vi "DisplayPanel.vi"() -> ()   [LabVIEW 2013]
uses:
  MvLVLib/MvCameraControl.lvlib
  <vilib>/picture/picture.llb/imagedata.ctl
panel:
  out "GenTLDevInfoArray":T1(array[cluster])
  out "GenTLIfInfoArray":T2(array[cluster])
  in  "Refresh Interaces":bool
  in  "Interface List":u16(ring) items=["[GenTL] GEVMV-GE1004-K88888888-100"]
  in  "pConvertInfo In":T3
  out "PixelFormat":u32
  out "handle out":u64
  in  "handle":u64
  in  "Rectangle":T4
  in  "image data":T5 caption="图像数据"
  out "Picture":picture
  out "PayloadSize":u32
  out "pFrameInfoEx out":T6
  out "nHeight":u32
  out "nWidth":u32
  out "Acquisision Flag":bool
  in  "Trigger Mode":bool
  in  "Continuous":bool
  out "打开标志":bool
  in  "stop":bool
  in  "Trigger Once":bool
  in  "Stop":bool
  in  "Start":bool
  in  "Open Device":bool
  in  "Close Device":bool
  in  "error in (no error) 2":errorcluster caption="错误输入（无错误）"
  in  "Refresh Devices":bool
  in  "Device List":u16(ring) items=["[GenTL]  MV-CA050-20GM(00598551000)"]
  # "Initialize"
  # "Acquisition"
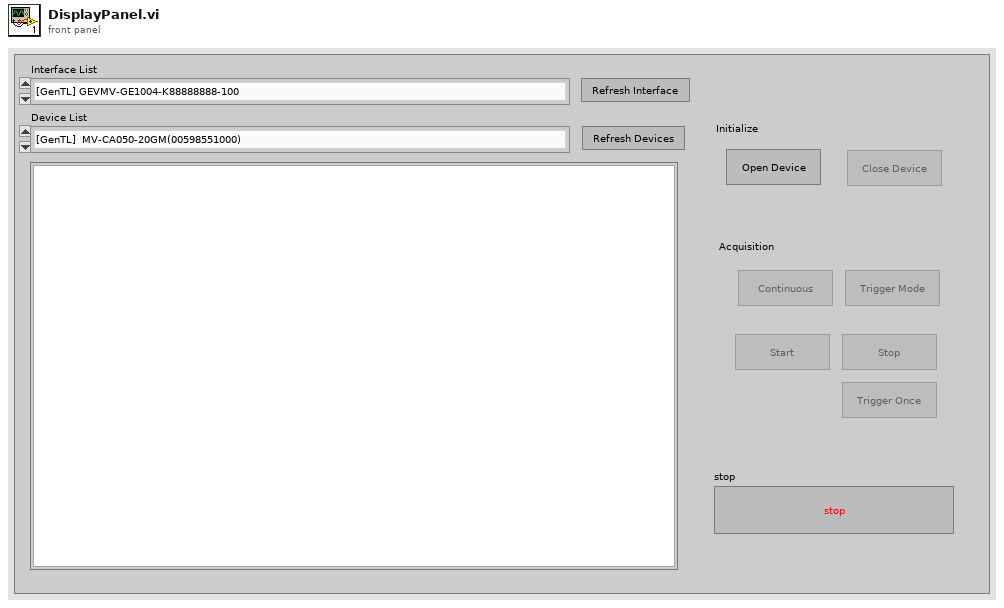
[diagram p1: front panel]
types:
  T1 = cluster{"chInterfaceID":string, "chDeviceID":string, "chVendorName":string, "chModelName":string, "chTLType":string, "chDisplayName":string, "chUserDefinedName":string, "chSerialNumber":string, "chDeviceVersion":string, "nCtiIndex":u32, "nReserved[0]":u32, "nReserved[1]":u32, "nReserved[2]":u32, "nReserved[3]":u32, "nReserved[4]":u32, "nReserved[5]":u32, "nReserved[6]":u32, "nReserved[7]":u32}[]
  T2 = cluster{"chInterfaceID":string, "chTLType":string, "chDisplayName":string, "nCtiIndex":u32, "nReserved[0]":u32, "nReserved[1]":u32, "nReserved[2]":u32, "nReserved[3]":u32, "nReserved[4]":u32, "nReserved[5]":u32, "nReserved[6]":u32, "nReserved[7]":u32}[]
  T3 = cluster{"nWidth":u16, "nHeight":u16, "enSrcPixelType":u32, "nSrcDataLen":u32, "enDstPixelType":u32, "nDstLen":u32, "nDstBufferSize":u32, "nRes0":u32, "nRes1":u32, "nRes2":u32, "nRes3":u32}
  T4 = cluster{"left":i16, "top":i16, "right":i16, "bottom":i16}
  T5 = typedef "imagedata.ctl" = cluster{"image type":i32, "image depth":i32, "image":u8[], "mask":u8[], "colors":u32[], "Rectangle":cluster{"left":i16, "top":i16, "right":i16, "bottom":i16}}
  T6 = cluster{"nWidth":u16, "nHeight":u16, "enPixelType":i32, "nFrameNum":u32, "nDevTimeStampHigh":u32, "nDevTimeStampLow":u32, "nReserved0":u32, "nHostTimeStamp":i64, "nFrameLen":u32, "nSecondCount]":u32, "nCycleCount":u32, "nCycleOffset":u32, "fGain":u32, "fExposureTime":u32, "nAverageBrightness":u32, "nRed":u32, "nGreen":u32, "nBlue":u32, "nFrameCounter":u32, "nTriggerIndex":u32, "nInput":u32, "nOutput":u32, "nOffsetX":u32, "nOffsetY":u32, "nReserved[0]":u32, "nReserved[1]":u32, "nReserved[2]":u32, "nReserved[3]":u32, "nReserved[4]":u32, "nReserved[5]":u32, "nReserved[6]":u32, "nReserved[7]":u32, "nReserved[8]":u32, "nReserved[9]":u32, "nReserved[10]":u32, "nReserved[11]":u32, "nReserved[12]":u32, "nReserved[13]":u32, "nReserved[14] 10":u32, "nReserved[15] 11":u32, "nReserved[16] 12":u32, "nReserved[17] 13":u32, "nReserved[18] 14":u32, "nReserved[19] 15":u32, "nReserved[20] 16":u32, "nReserved[21] 17":u32, "nReserved[22] 18":u32, "nReserved[23] 19":u32, "nReserved[24] 20":u32, "nReserved[25] 21":u32, "nReserved[26] 22":u32, "nReserved[27] 23":u32, "nReserved[28] 24":u32, "nReserved[29] 25":u32, "nReserved[30] 26":u32, "nReserved[31] 27":u32, "nReserved[32] 28":u32, "nReserved[33] 29":u32, "nReserved[34] 30":u32, "nReserved[35] 31":u32, "nReserved[36] 32":u32, "nReserved[37] 33":u32, "nReserved[38] 34":u32, "nReserved[39] 35":u32, "nReserved[40] 36":u32}
  T7 = enum8{"Enabled", "Disabled", "Disabled and Grayed Out"}
  T8 = cluster{"chInterfaceID":string, "chTLType":string, "chDisplayName":string, "nCtiIndex":u32, "nReserved[0]":u32, "nReserved[1]":u32, "nReserved[2]":u32, "nReserved[3]":u32, "nReserved[4]":u32, "nReserved[5]":u32, "nReserved[6]":u32, "nReserved[7]":u32}
  T9 = cluster{"chInterfaceID":string, "chDeviceID":string, "chVendorName":string, "chModelName":string, "chTLType":string, "chDisplayName":string, "chUserDefinedName":string, "chSerialNumber":string, "chDeviceVersion":string, "nCtiIndex":u32, "nReserved[0]":u32, "nReserved[1]":u32, "nReserved[2]":u32, "nReserved[3]":u32, "nReserved[4]":u32, "nReserved[5]":u32, "nReserved[6]":u32, "nReserved[7]":u32}
  T10 = cluster{"nCurValue":u32, "nMax":u32, "nMin":u32, "nInc":u32, "nReserved[0]":u32, "nReserved[1]":u32, "nReserved[2]":u32, "nReserved[3]":u32}
  T11 = cluster{"nCurValue":u32, "nSupportedNum":u32, "nSupportValue":u32[], "nReserved[0]":u32, "nReserved[1]":u32, "nReserved[2]":u32, "nReserved[3]":u32}
  T12 = cluster{"nWidth":u32, "nHeight":u32, "enSrcPixelType":u32, "nSrcDataLen":u32, "enDstPixelType":u32, "nDstLen":u32, "nDstBufferSize":u32, "nRes0":u32, "nRes1":u32, "nRes2":u32, "nRes3":u32}
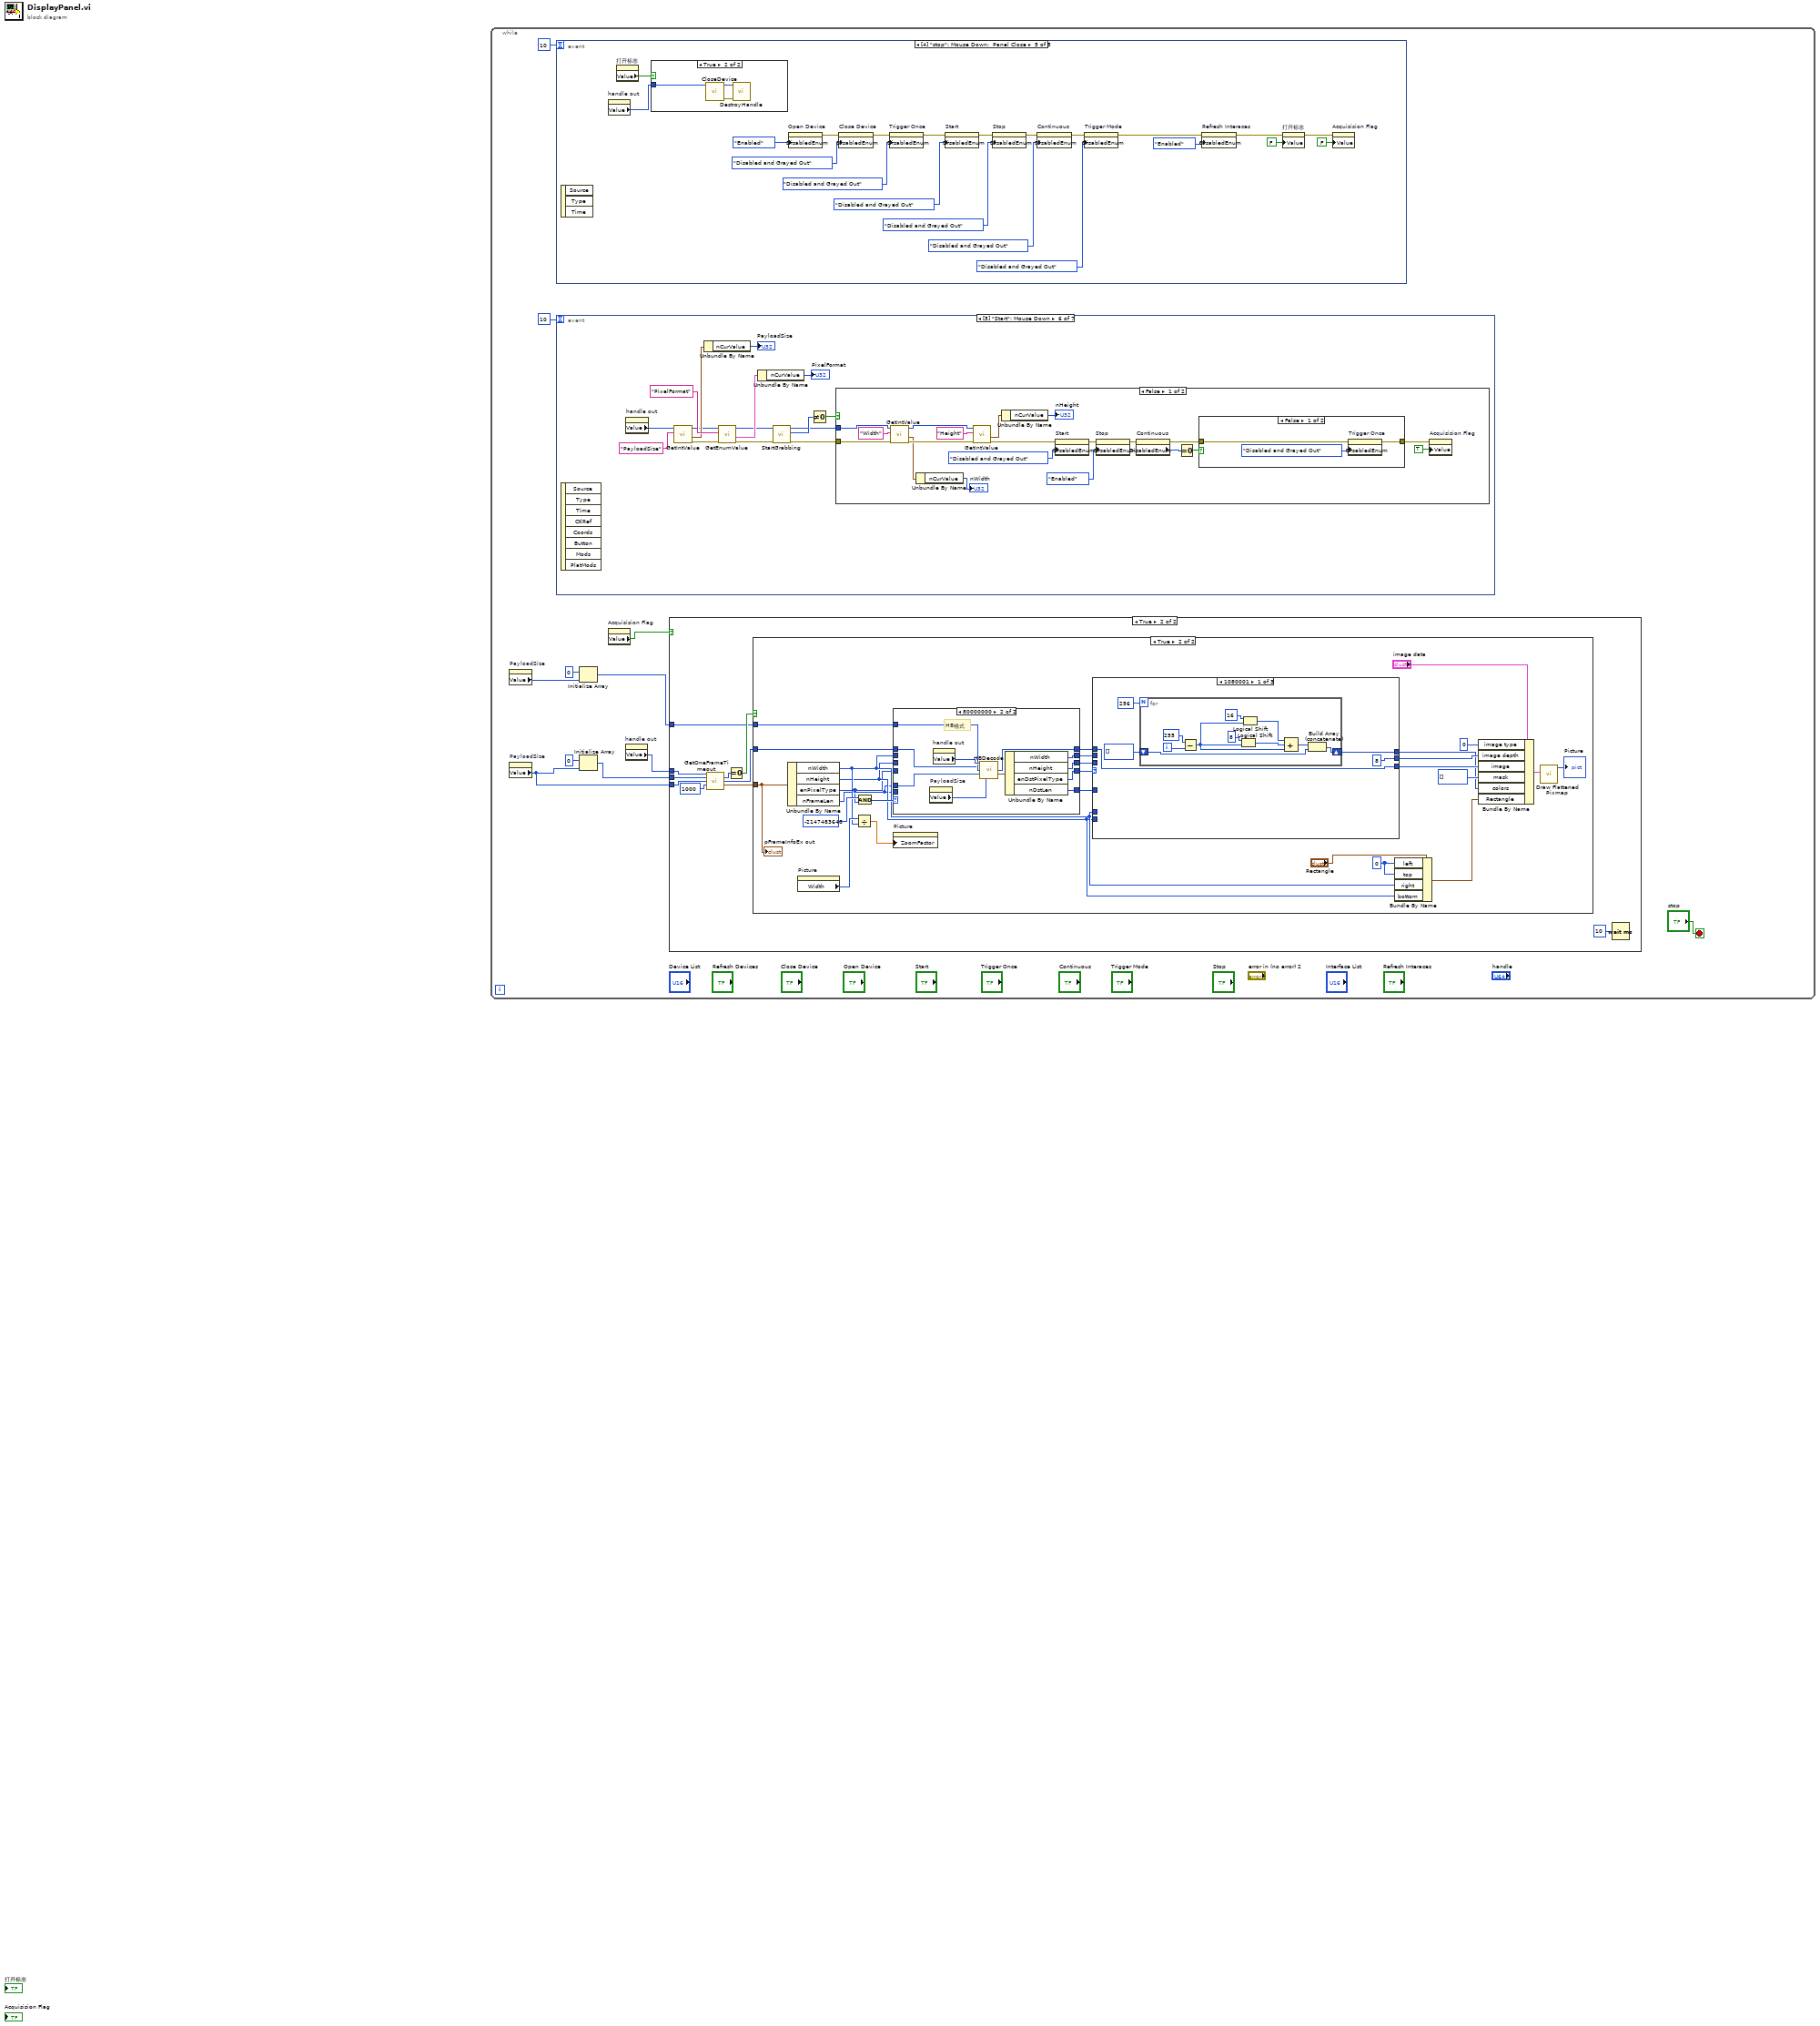
[diagram p0: block diagram]
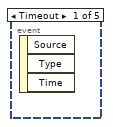
[diagram p2: hidden frame]
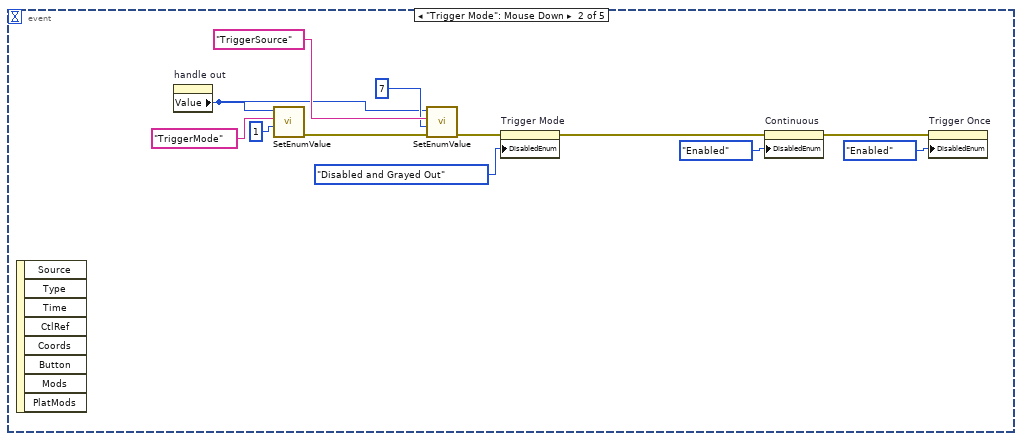
[diagram p3: hidden frame]
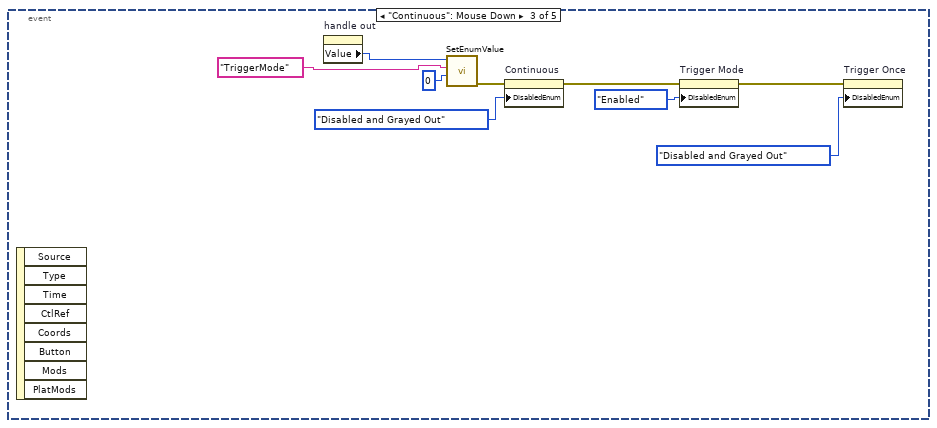
[diagram p4: hidden frame]
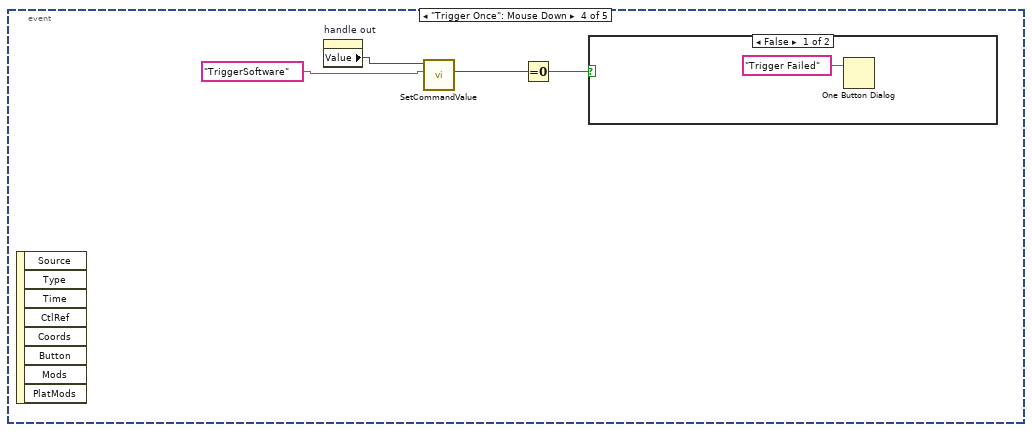
[diagram p5: hidden frame]
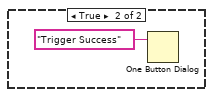
[diagram p6: hidden frame]
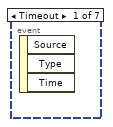
[diagram p8: hidden frame]
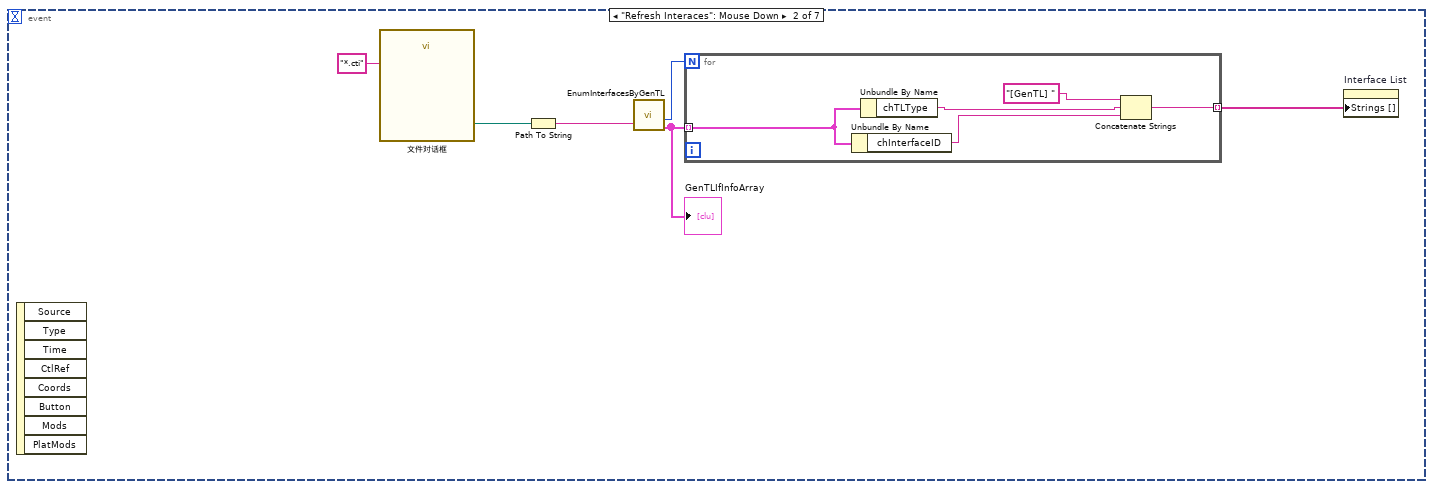
[diagram p9: hidden frame]
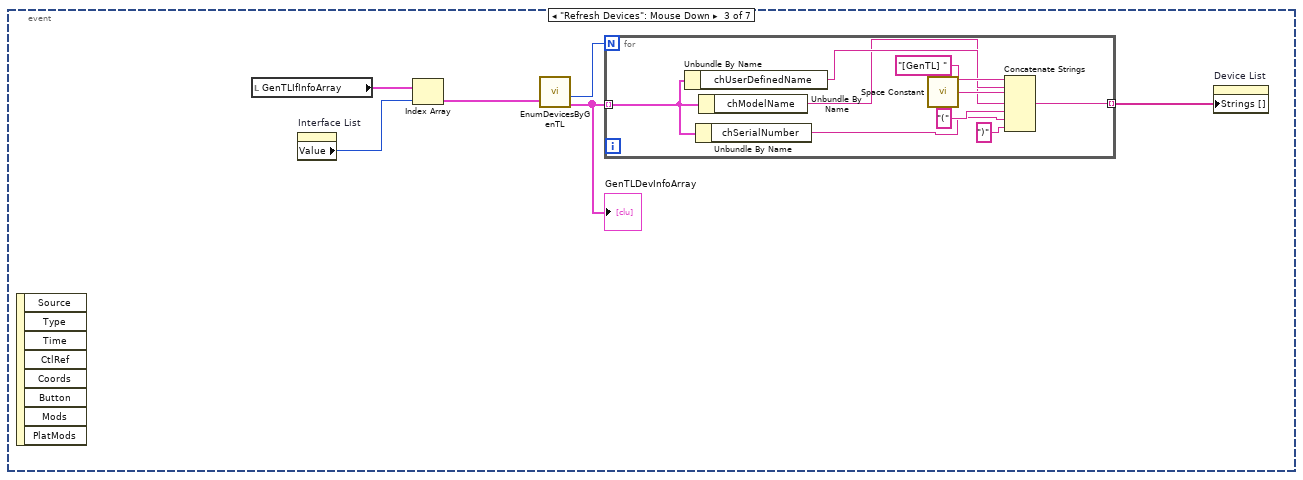
[diagram p10: hidden frame]
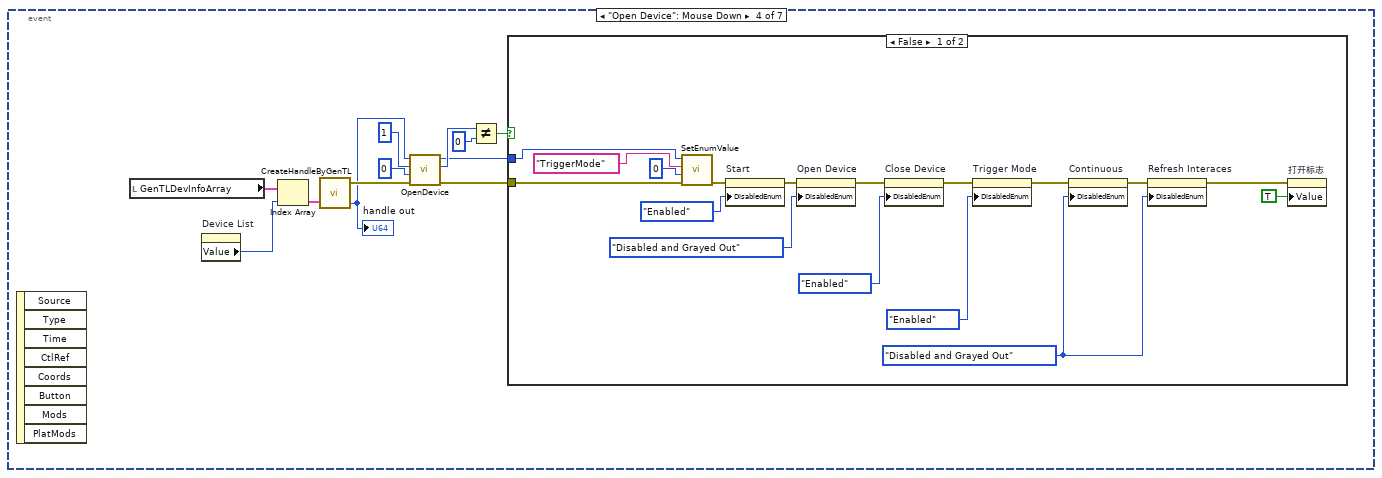
[diagram p11: hidden frame]
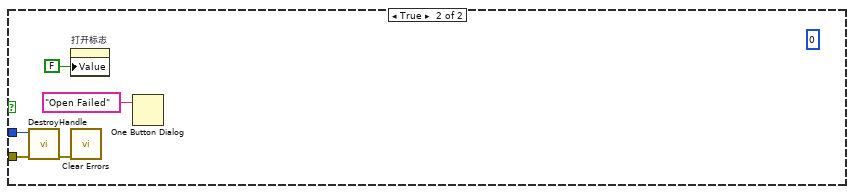
[diagram p12: hidden frame]
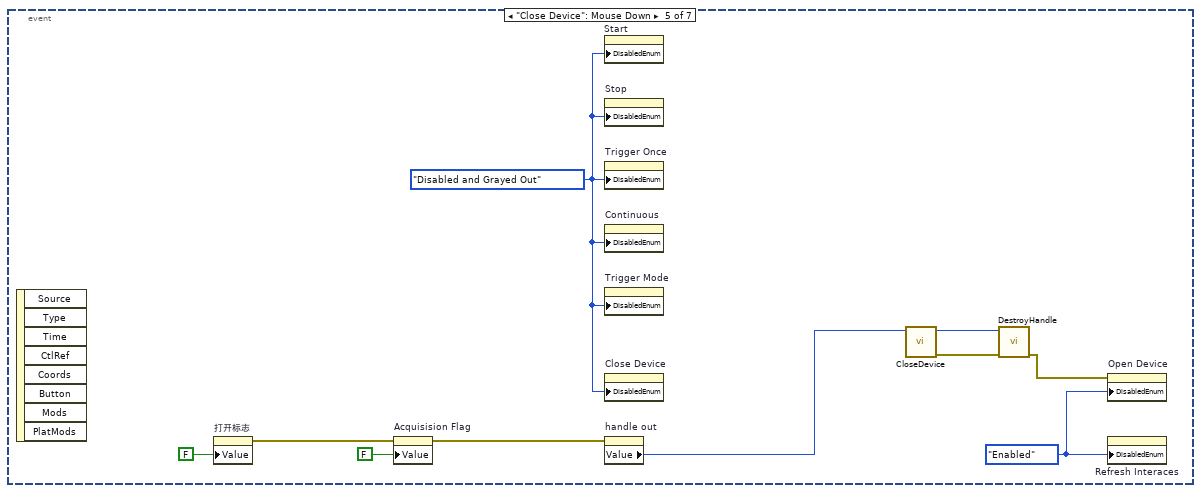
[diagram p13: hidden frame]
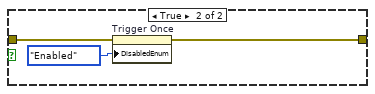
[diagram p14: hidden frame]
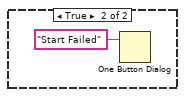
[diagram p15: hidden frame]
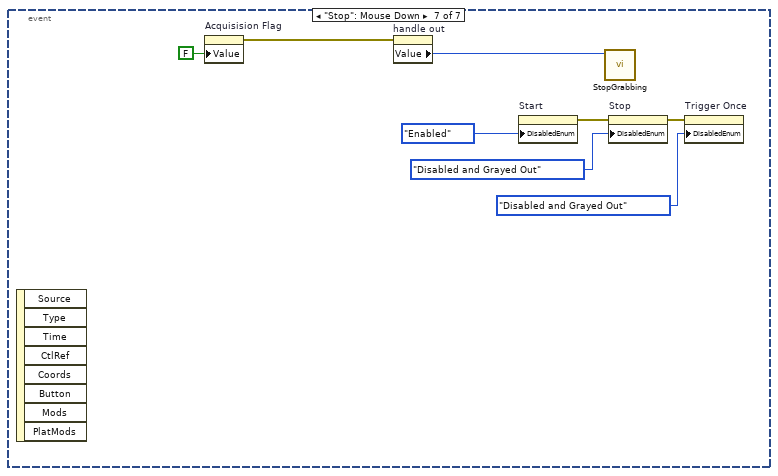
[diagram p16: hidden frame]
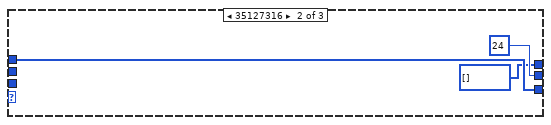
[diagram p20: hidden frame]
diagram:
  n1 = while {
    stop <- "stop" stop-if-true
    n2 = property on="PayloadSize" class="DigNum (strict)"() -> ("Value"=w5:u32)  [unwired: 2 in, 2 out]
    n3 = property on="PayloadSize" class="DigNum (strict)"() -> ("Value"=w6:u32)  [unwired: 2 in, 2 out]
    n4 = event shown="[4] \"stop\": Mouse Down;  Panel Close" {
      selector: _ -> [_ _ _ _ _]
      dyn-events: _ -> [_ _ _ _ _]
      timeout: 10 -> [_ _ _ _ _]
      event Timeout {
        n5 = event-data() -> ()  [unwired: 1 in, 3 out]
      }
      event "Trigger Mode": Mouse Down {
        n6 = event-data() -> ()  [unwired: 1 in, 8 out]
        n7 = property on="handle out" class="DigNum (strict)"() -> ("Value"=w12:u64)  [unwired: 2 in, 2 out]
        n8 = call "SetEnumValue.vi"("nValue"=u32 1, "strKey"="TriggerMode", "handle"=w12) -> ("error out"=w18:errorcluster)  [unwired: 6 in, 2 out]
        n9 = call "SetEnumValue.vi"("error in (no error)"=w18, "nValue"=u32 7, "strKey"="TriggerSource", "handle"=w12) -> ("error out"=w17:errorcluster)  [unwired: 5 in, 2 out]
        n10 = property on="Trigger Mode" class="Bool"(error in=w17, "DisabledEnum"=T7."Disabled and Grayed Out" ("禁用")) -> (error out=w16:errorcluster)  [unwired: 1 in, 1 out]
        n11 = property on="Continuous" class="Bool"(error in=w16, "DisabledEnum"=T7."Enabled" ("禁用")) -> (error out=w14:errorcluster)  [unwired: 1 in, 1 out]
        n12 = property on="Trigger Once" class="Bool"(error in=w14, "DisabledEnum"=T7."Enabled" ("禁用")) -> ()  [unwired: 1 in, 2 out]
      }
      event "Continuous": Mouse Down {
        n13 = event-data() -> ()  [unwired: 1 in, 8 out]
        n14 = property on="handle out" class="DigNum (strict)"() -> ("Value"=w24:u64)  [unwired: 2 in, 2 out]
        n15 = call "SetEnumValue.vi"("nValue"=u32 0, "strKey"="TriggerMode", "handle"=w24) -> ("error out"=w25:errorcluster)  [unwired: 6 in, 2 out]
        n16 = property on="Continuous" class="Bool"(error in=w25, "DisabledEnum"=T7."Disabled and Grayed Out" ("禁用")) -> (error out=w29:errorcluster)  [unwired: 1 in, 1 out]
        n17 = property on="Trigger Mode" class="Bool"(error in=w29, "DisabledEnum"=T7."Enabled" ("禁用")) -> (error out=w27:errorcluster)  [unwired: 1 in, 1 out]
        n18 = property on="Trigger Once" class="Bool"(error in=w27, "DisabledEnum"=T7."Disabled and Grayed Out" ("禁用")) -> ()  [unwired: 1 in, 2 out]
      }
      event "Trigger Once": Mouse Down {
        n19 = event-data() -> ()  [unwired: 1 in, 8 out]
        n20 = property on="handle out" class="DigNum (strict)"() -> ("Value"=w33:u64)  [unwired: 2 in, 2 out]
        n21 = call "SetCommandValue.vi"("strValue"="TriggerSoftware", "handle"=w33) -> ("function return"=w35:i32)  [unwired: 7 in, 2 out]
        n22 = Equal To 0?(x=w35) -> (x = 0?=w34:bool)
        n23 = case shown="False" w34 {
          frame False {
            n24 = One Button Dialog(message="Trigger Failed") -> ()  [unwired: 1 in, 1 out]
          }
          frame True {
            n25 = One Button Dialog(message="Trigger Success") -> ()  [unwired: 1 in, 1 out]
          }
        }
      }
      event "stop": Mouse Down; Panel Close {
        n26 = event-data() -> ()  [unwired: 1 in, 3 out]
        n27 = property on="handle out" class="DigNum (strict)"() -> ("Value"=w39:u64)  [unwired: 2 in, 2 out]
        n28 = property on="打开标志" class="Bool (strict)"() -> ("Value"=w46:bool)  [unwired: 2 in, 2 out]
        n29 = case shown="True" w46 {
          tunnel: w39 -> [_ w61]
          frame False {
          }
          frame True {
            n30 = call "CloseDevice.vi"("handle"=w61) -> ("error out"=w62:errorcluster, "handle out"=w60:u64)  [unwired: 8 in, 1 out]
            n31 = call "DestroyHandle.vi"("error in (no error)"=w62, "handle"=w60) -> ()  [unwired: 8 in, 2 out]
          }
        }
        n32 = property on="Open Device" class="Bool"("DisabledEnum"=T7."Enabled" ("禁用")) -> (error out=w54:errorcluster)  [unwired: 2 in, 1 out]
        n33 = property on="Close Device" class="Bool"(error in=w54, "DisabledEnum"=T7."Disabled and Grayed Out" ("禁用")) -> (error out=w53:errorcluster)  [unwired: 1 in, 1 out]
        n34 = property on="Trigger Once" class="Bool"(error in=w53, "DisabledEnum"=T7."Disabled and Grayed Out" ("禁用")) -> (error out=w52:errorcluster)  [unwired: 1 in, 1 out]
        n35 = property on="Start" class="Bool"(error in=w52, "DisabledEnum"=T7."Disabled and Grayed Out" ("禁用")) -> (error out=w51:errorcluster)  [unwired: 1 in, 1 out]
        n36 = property on="Stop" class="Bool"(error in=w51, "DisabledEnum"=T7."Disabled and Grayed Out" ("禁用")) -> (error out=w50:errorcluster)  [unwired: 1 in, 1 out]
        n37 = property on="Continuous" class="Bool"(error in=w50, "DisabledEnum"=T7."Disabled and Grayed Out" ("禁用")) -> (error out=w48:errorcluster)  [unwired: 1 in, 1 out]
        n38 = property on="Trigger Mode" class="Bool"(error in=w48, "DisabledEnum"=T7."Disabled and Grayed Out" ("禁用")) -> (error out=w41:errorcluster)  [unwired: 1 in, 1 out]
        n39 = property on="Refresh Interaces" class="Bool"(error in=w41, "DisabledEnum"=T7."Enabled" ("禁用")) -> (error out=w40:errorcluster)  [unwired: 1 in, 1 out]
        n40 = property on="打开标志" class="Bool (strict)"(error in=w40, "Value"=FALSE ("打开标志")) -> (error out=w43:errorcluster)  [unwired: 1 in, 1 out]
        n41 = property on="Acquisision Flag" class="Bool (strict)"(error in=w43, "Value"=FALSE ("采集标志")) -> ()  [unwired: 1 in, 2 out]
      }
    }
    n42 = event shown="[5] \"Start\": Mouse Down" {
      selector: _ -> [_ _ _ _ _ _ _]
      dyn-events: _ -> [_ _ _ _ _ _ _]
      timeout: 10 -> [_ _ _ _ _ _ _]
      event Timeout {
        n43 = event-data() -> ()  [unwired: 1 in, 3 out]
      }
      event "Refresh Interaces": Mouse Down {
        n44 = event-data() -> ()  [unwired: 1 in, 8 out]
        n45 = call "文件对话框"("pattern (all files)"="*.cti") -> ("selected path"=w67:path)  [unwired: 11 in, 3 out]
        n46 = Path To String(path=w67) -> (string=w66:string)
        n47 = call "EnumInterfacesByGenTL.vi"("strGenTLPath"=w66) -> ("nInterfaceNum"=w64:u32, "pGenTLIfInfoArray"=w65:T2)  [unwired: 1 in, 2 out]
        "GenTLIfInfoArray" <- w65
        n48 = for {
          N: w64 -> [_]
          tunnel: [w73] -> w63 mode=indexing
          tunnel: w65 -> [w70] mode=indexing
          n49 = Unbundle By Name(w70) -> ("chInterfaceID"=w71:string)
          n50 = Unbundle By Name(w70) -> ("chTLType"=w69:string)
          n51 = Concatenate Strings("[GenTL] " ("字符串"), w69, w71) -> (w73:string)
        }
        n52 = property on="Interface List" class="Ring (strict)"("Strings []"=w63) -> ()  [unwired: 2 in, 2 out]
      }
      event "Refresh Devices": Mouse Down {
        n53 = event-data() -> ()  [unwired: 1 in, 8 out]
        n54 = local read "GenTLIfInfoArray"() -> (w77:T2)
        n55 = property on="Interface List" class="Ring (strict)"() -> ("Value"=w78:u16)  [unwired: 2 in, 2 out]
        n56 = Index Array(array=w77, index=w78) -> (element=w76:T8)
        n57 = call "EnumDevicesByGenTL.vi"("pIFInfo"=w76) -> ("nDeviceNum"=w75:u32, "pGenTLDevInfoArray"=w74:T1)  [unwired: 1 in, 2 out]
        "GenTLDevInfoArray" <- w74
        n58 = for {
          N: w75 -> [_]
          tunnel: [w85] -> w79 mode=indexing
          tunnel: w74 -> [w83] mode=indexing
          n59 = Unbundle By Name(w83) -> ("chUserDefinedName"=w82:string)
          n60 = Unbundle By Name(w83) -> ("chSerialNumber"=w80:string)
          n61 = Unbundle By Name(w83) -> ("chModelName"=w81:string)
          n62 = call <vilib>:"Space Constant.vi"() -> ("String"=w88:string)
          n63 = Concatenate Strings("[GenTL] " ("字符串"), w82, w88, w81, "(" ("字符串"), w80, ")" ("字符串")) -> (w85:string)
        }
        n64 = property on="Device List" class="Ring (strict)"("Strings []"=w79) -> ()  [unwired: 2 in, 2 out]
      }
      event "Open Device": Mouse Down {
        n65 = event-data() -> ()  [unwired: 1 in, 8 out]
        n66 = local read "GenTLDevInfoArray"() -> (w89:T1)
        n67 = property on="Device List" class="Ring (strict)"() -> ("Value"=w93:u16)  [unwired: 2 in, 2 out]
        n68 = Index Array(array=w89, index=w93) -> (element=w90:T9)
        n69 = call "CreateHandleByGenTL.vi"("pDevInfo"=w90) -> ("error out"=w92:errorcluster, "handle"=w91:u64)  [unwired: 1 in, 1 out]
        "handle out" <- w91
        n70 = call "OpenDevice.vi"("error in (no error)"=w92, "nSwitchoverKey"=u16 0, "nAccessMode"=u32 1, "handle"=w91) -> ("error out"=w96:errorcluster, "return"=w95:i32, "handle out"=w94:u64)  [unwired: 5 in]
        n71 = Not Equal?(x=w95, y=0) -> (x != y?=w99:bool)
        n72 = case shown="False" w99 {
          tunnel: w94 -> [w104 w120]
          tunnel: w96 -> [w105 w118]
          frame False {
            w103 = T7."Disabled and Grayed Out" ("禁用")
            n73 = call "SetEnumValue.vi"("error in (no error)"=w105, "nValue"=u32 0, "strKey"="TriggerMode", "handle"=w104) -> ("error out"=w114:errorcluster)  [unwired: 5 in, 2 out]
            n74 = property on="Start" class="Bool"(error in=w114, "DisabledEnum"=T7."Enabled" ("禁用")) -> (error out=w112:errorcluster)  [unwired: 1 in, 1 out]
            n75 = property on="Open Device" class="Bool"(error in=w112, "DisabledEnum"=T7."Disabled and Grayed Out" ("禁用")) -> (error out=w111:errorcluster)  [unwired: 1 in, 1 out]
            n76 = property on="Close Device" class="Bool"(error in=w111, "DisabledEnum"=T7."Enabled" ("禁用")) -> (error out=w108:errorcluster)  [unwired: 1 in, 1 out]
            n77 = property on="Trigger Mode" class="Bool"(error in=w108, "DisabledEnum"=T7."Enabled" ("禁用")) -> (error out=w107:errorcluster)  [unwired: 1 in, 1 out]
            n78 = property on="Continuous" class="Bool"(error in=w107, "DisabledEnum"=w103) -> (error out=w102:errorcluster)  [unwired: 1 in, 1 out]
            n79 = property on="Refresh Interaces" class="Bool"(error in=w102, "DisabledEnum"=w103) -> (error out=w101:errorcluster)  [unwired: 1 in, 1 out]
            n80 = property on="打开标志" class="Bool (strict)"(error in=w101, "Value"=TRUE ("布尔")) -> ()  [unwired: 1 in, 2 out]
          }
          frame True {
            (unwired) u64 0 ("handle")
            n81 = call "DestroyHandle.vi"("error in (no error)"=w118, "handle"=w120) -> ("error out"=w119:errorcluster)  [unwired: 8 in, 1 out]
            n82 = property on="打开标志" class="Bool (strict)"("Value"=FALSE) -> ()  [unwired: 2 in, 2 out]
            n83 = call <vilib>:"Clear Errors.vi"("error in (no error)"=w119) -> ()  [unwired: 5 in, 2 out]
            n84 = One Button Dialog(message="Open Failed") -> ()  [unwired: 1 in, 1 out]
          }
        }
      }
      event "Close Device": Mouse Down {
        w123 = T7."Enabled" ("禁用")
        w124 = T7."Disabled and Grayed Out" ("禁用")
        n85 = event-data() -> ()  [unwired: 1 in, 8 out]
        n86 = property on="打开标志" class="Bool (strict)"("Value"=FALSE ("打开标志")) -> (error out=w131:errorcluster)  [unwired: 2 in, 1 out]
        n87 = property on="Acquisision Flag" class="Bool (strict)"(error in=w131, "Value"=FALSE ("采集标志")) -> (error out=w125:errorcluster)  [unwired: 1 in, 1 out]
        n88 = property on="Start" class="Bool"("DisabledEnum"=w124) -> ()  [unwired: 2 in, 2 out]
        n89 = property on="Stop" class="Bool"("DisabledEnum"=w124) -> ()  [unwired: 2 in, 2 out]
        n90 = property on="Trigger Once" class="Bool"("DisabledEnum"=w124) -> ()  [unwired: 2 in, 2 out]
        n91 = property on="Continuous" class="Bool"("DisabledEnum"=w124) -> ()  [unwired: 2 in, 2 out]
        n92 = property on="Trigger Mode" class="Bool"("DisabledEnum"=w124) -> ()  [unwired: 2 in, 2 out]
        n93 = property on="Close Device" class="Bool"("DisabledEnum"=w124) -> ()  [unwired: 2 in, 2 out]
        n94 = property on="handle out" class="DigNum (strict)"(error in=w125) -> ("Value"=w126:u64)  [unwired: 1 in, 2 out]
        n95 = call "CloseDevice.vi"("handle"=w126) -> ("error out"=w129:errorcluster, "handle out"=w127:u64)  [unwired: 8 in, 1 out]
        n96 = call "DestroyHandle.vi"("error in (no error)"=w129, "handle"=w127) -> ("error out"=w128:errorcluster)  [unwired: 8 in, 1 out]
        n97 = property on="Open Device" class="Bool"(error in=w128, "DisabledEnum"=w123) -> ()  [unwired: 1 in, 2 out]
        n98 = property on="Refresh Interaces" class="Bool"("DisabledEnum"=w123) -> ()  [unwired: 2 in, 2 out]
      }
      event "Start": Mouse Down {
        n99 = event-data() -> ()  [unwired: 1 in, 8 out]
        n100 = property on="handle out" class="DigNum (strict)"() -> ("Value"=w133:u64)  [unwired: 2 in, 2 out]
        n101 = call "GetIntValue.vi"("strKey"="PayloadSize", "handle"=w133) -> ("error out"=w143:errorcluster, "pIntValue out"=w139:T10, "handle out"=w136:u64)  [unwired: 6 in, 1 out]
        n102 = Unbundle By Name(w139) -> ("nCurValue"=→"PayloadSize":u32)
        n103 = call "GetEnumValue.vi"("error in (no error)"=w143, "strKey"="PixelFormat", "handle"=w136) -> ("error out"=w142:errorcluster, "pEnumValue out"=w144:T11, "handle out"=w135:u64)  [unwired: 5 in, 1 out]
        n104 = Unbundle By Name(w144) -> ("nCurValue"=→"PixelFormat":u32)
        n105 = call "StartGrabbing.vi"("error in (no error)"=w142, "handle"=w135) -> ("error out"=w141:errorcluster, "function return"=w147:i32, "handle out"=w134:u64)  [unwired: 7 in]
        n106 = Not Equal To 0?(x=w147) -> (x != 0?=w146:bool)
        n107 = case shown="False" w146 {
          tunnel: w141 -> [w150 _]
          tunnel: w134 -> [w149 _]
          frame False {
            n108 = call "GetIntValue.vi"("error in (no error)"=w150, "strKey"="Width", "handle"=w149) -> ("error out"=w157:errorcluster, "pIntValue out"=w151:T10, "handle out"=w148:u64)  [unwired: 5 in, 1 out]
            n109 = Unbundle By Name(w151) -> ("nCurValue"=→"nWidth":u32)
            n110 = call "GetIntValue.vi"("error in (no error)"=w157, "strKey"="Height", "handle"=w148) -> ("error out"=w156:errorcluster, "pIntValue out"=w154:T10)  [unwired: 5 in, 2 out]
            n111 = Unbundle By Name(w154) -> ("nCurValue"=→"nHeight":u32)
            n112 = property on="Start" class="Bool"(error in=w156, "DisabledEnum"=T7."Disabled and Grayed Out" ("禁用")) -> (error out=w166:errorcluster)  [unwired: 1 in, 1 out]
            n113 = property on="Stop" class="Bool"(error in=w166, "DisabledEnum"=T7."Enabled" ("禁用")) -> (error out=w152:errorcluster)  [unwired: 1 in, 1 out]
            n114 = property on="Continuous" class="Bool"(error in=w152) -> (error out=w162:errorcluster, "DisabledEnum"=w163:T7)  [unwired: 1 in, 1 out]
            n115 = Equal To 0?(x=w163) -> (x = 0?=w164:bool)
            n116 = case shown="False" w164 {
              tunnel: w162 -> [w169 w172]
              tunnel: [w168 w171] -> w161
              frame False {
                n117 = property on="Trigger Once" class="Bool"(error in=w169, "DisabledEnum"=T7."Disabled and Grayed Out" ("禁用")) -> (error out=w168:errorcluster)  [unwired: 1 in, 1 out]
              }
              frame True {
                n118 = property on="Trigger Once" class="Bool"(error in=w172, "DisabledEnum"=T7."Enabled" ("禁用")) -> (error out=w171:errorcluster)  [unwired: 1 in, 1 out]
              }
            }
            n119 = property on="Acquisision Flag" class="Bool (strict)"(error in=w161, "Value"=TRUE ("采集标志")) -> ()  [unwired: 1 in, 2 out]
          }
          frame True {
            n120 = One Button Dialog(message="Start Failed") -> ()  [unwired: 1 in, 1 out]
          }
        }
      }
      event "Stop": Mouse Down {
        n121 = event-data() -> ()  [unwired: 1 in, 8 out]
        n122 = property on="Acquisision Flag" class="Bool (strict)"("Value"=FALSE ("采集标志")) -> (error out=w175:errorcluster)  [unwired: 2 in, 1 out]
        n123 = property on="handle out" class="DigNum (strict)"(error in=w175) -> ("Value"=w176:u64)  [unwired: 1 in, 2 out]
        n124 = property on="Start" class="Bool"("DisabledEnum"=T7."Enabled" ("禁用")) -> (error out=w178:errorcluster)  [unwired: 2 in, 1 out]
        n125 = call "StopGrabbing.vi"("handle"=w176) -> ()  [unwired: 8 in, 3 out]
        n126 = property on="Stop" class="Bool"(error in=w178, "DisabledEnum"=T7."Disabled and Grayed Out" ("禁用")) -> (error out=w177:errorcluster)  [unwired: 1 in, 1 out]
        n127 = property on="Trigger Once" class="Bool"(error in=w177, "DisabledEnum"=T7."Disabled and Grayed Out" ("禁用")) -> ()  [unwired: 1 in, 2 out]
      }
    }
    n128 = Initialize Array(u8 0 ("元素"), w5) -> (w4:u8[])
    n129 = Initialize Array(u8 0 ("元素"), w6) -> (w7:u8[])
    n130 = property on="Acquisision Flag" class="Bool (strict)"() -> ("Value"=w11:bool)  [unwired: 2 in, 2 out]
    n131 = property on="handle out" class="DigNum (strict)"() -> ("Value"=w9:u64)  [unwired: 2 in, 2 out]
    n132 = case shown="True" w11 {
      tunnel: w9 -> [_ w189]
      tunnel: w7 -> [_ w188]
      tunnel: w6 -> [_ w187]
      tunnel: w4 -> [_ w183]
      frame False {
      }
      frame True {
        n133 = call "GetOneFrameTimeout.vi"("handle"=w189, "pData"=w188, "nDataSize"=w187, "nMsec"=1000) -> ("function return"=w186:i32, "pData Out"=w185:u8[], "pFrameInfoEx out"=w184:T6)  [unwired: 7 in, 2 out]
        n134 = Equal To 0?(x=w186) -> (x = 0?=w191:bool)
        n135 = case shown="True" w191 {
          tunnel: w185 -> [_ w202]
          tunnel: w184 -> [_ w206]
          tunnel: w183 -> [_ w203]
          frame False {
          }
          frame True {
            w216 = i16 0 ("left")
            n136 = Unbundle By Name(w206) -> ("nWidth"=w201:u16, "nHeight"=w200:u16, "enPixelType"=w193:i32, "nFrameLen"=w199:u32)
            n137 = property on="Picture" class="Pict"() -> ("Width"=w211:u32)  [unwired: 2 in, 2 out]
            n138 = Divide(x=w211, y=w201) -> (x/y=w210:dbl)
            n139 = Compound Arithmetic op=AND(-2147483648 ("value"), w193) -> (w204:i32)
            n140 = case shown="80000000" w204 {
              tunnel: [w224 w232] -> w198
              tunnel: [w223 w231] -> w197
              tunnel: [w222 w230] -> w196
              tunnel: [w220 w229] -> w194
              tunnel: [w221 w228] -> w195
              tunnel: w203 -> [_ w227]
              tunnel: w202 -> [w224 w226]
              tunnel: w199 -> [_ w225]
              tunnel: w201 -> [w223 _]
              tunnel: w200 -> [w222 _]
              tunnel: w199 -> [w221 _]
              tunnel: w193 -> [w220 _]
              frame Default {
              }
              frame -2147483648 {
                # "HB格式"
                n141 = property on="PayloadSize" class="DigNum (strict)"() -> ("Value"=w234:u32)  [unwired: 2 in, 2 out]
                n142 = property on="handle out" class="DigNum (strict)"() -> ("Value"=w235:u64)  [unwired: 2 in, 2 out]
                n143 = call "HBDecode.vi"("handle"=w235, "pSrcData"=w226, "pDstBuf In"=w227, "SrcDataLen"=w225, "DstBufferSize"=w234) -> ("pDstBuf Out"=w232:u8[], "pHBDecode Out"=w233:T12)  [unwired: 6 in, 3 out]
                n144 = Unbundle By Name(w233) -> ("nWidth"=w231:u32, "nHeight"=w230:u32, "enDstPixelType"=w229:u32, "nDstLen"=w228:u32)
              }
            }
            n145 = property on="Picture" class="Pict"("ZoomFactor"=w210) -> ()  [unwired: 2 in, 2 out]
            n146 = case shown="1080001" w194 {
              selector: w194 -> [_ _ w254]
              tunnel: w198 -> [w238 w253 w268]
              tunnel: w200 -> [_ _ w265]
              tunnel: w201 -> [_ _ w264]
              tunnel: [w238 w253 w258] -> w209
              tunnel: [8 24 24] -> w208
              tunnel: [w236 i32[] [] i32[] []] -> w207
              tunnel: w197 -> [_ _ w257]
              tunnel: w196 -> [_ _ w256]
              tunnel: w195 -> [_ _ w255]
              frame 17301505 {
                n147 = for {
                  N: 256 -> [_]
                  shift-right: [w245] -> w236
                  shift-left: i32[] [] ("数组") -> [w244]
                  i -> [w241]
                  n148 = Subtract(x=255, y=w241) -> (x-y=w242:i32)
                  n149 = Logical Shift(y=i16 8, x=w242) -> (x << y=w247:i32)
                  n150 = Logical Shift(y=16 ("x"), x=w242) -> (x << y=w248:i32)
                  n151 = Compound Arithmetic op=ADD(w248, w247, w242) -> (w246:i32)
                  n152 = Build Array (concatenate)(w246, w244) -> (w245:i32[])
                }
              }
              frame 35127316 {
              }
              frame Default {
                n153 = Compound Arithmetic op=MULTIPLY(w265, w264, u32 3 ("值")) -> (w262:u32)
                n154 = Bundle By Name(cluster="pConvertInfo In", "nWidth"=w257, "nHeight"=w256, "enSrcPixelType"=w254, "nSrcDataLen"=w255, "enDstPixelType"=u32 35127316, "nDstBufferSize"=w262) -> (w261:T3)
                n155 = property on="handle out" class="DigNum (strict)"() -> ("Value"=w269:u64)  [unwired: 2 in, 2 out]
                n156 = Initialize Array(u8 0 ("元素"), w262) -> (w267:u8[])
                n157 = call "ConvertPixelType.vi"("handle"=w269, "pSrcData"=w268, "pDstBuf In"=w267, "pConvertInfo In"=w261) -> ("pDstBuf Out"=w258:u8[])  [unwired: 7 in, 4 out]
              }
            }
            n158 = Bundle By Name(cluster="Rectangle", "left"=w216, "top"=w216, "right"=w201, "bottom"=w200) -> (w213:T4)
            n159 = Bundle By Name(cluster="image data", "image type"=0, "image depth"=w208, "image"=w209, "mask"=u8[] [], "colors"=w207, "Rectangle"=w213) -> (w212:T5)
            n160 = call <vilib>:"Draw Flattened Pixmap.vi"("image data"=w212) -> ("new picture"=→"Picture":picture)  [unwired: 8 in]
            "pFrameInfoEx out" <- w206
          }
        }
        n161 = Wait (ms)(milliseconds to wait=u32 10 ("等待时间（毫秒）")) -> ()  [unwired: 1 out]
      }
    }
  }
